vi "Set_Tips_Position_XY.vi"(8 "XYGraph输入":refnum<vi>, 9 "Offset":u8, 10 "Coords":T1, 11 "TipsRef":refnum<vi>) -> ()   [LabVIEW 2015]
uses:
  <vilib>/Utility/miscctls.llb/LVPoint32TypeDef.ctl
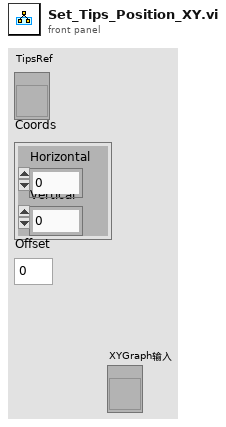
[diagram p1: front panel]
types:
  T1 = typedef "LVPoint32TypeDef.ctl" = cluster{"Horizontal":i32, "Vertical":i32}
  T2 = typedef "LVRectTypeDef.ctl" = cluster{"Left":i16, "Top":i16, "Right":i16, "Bottom":i16}
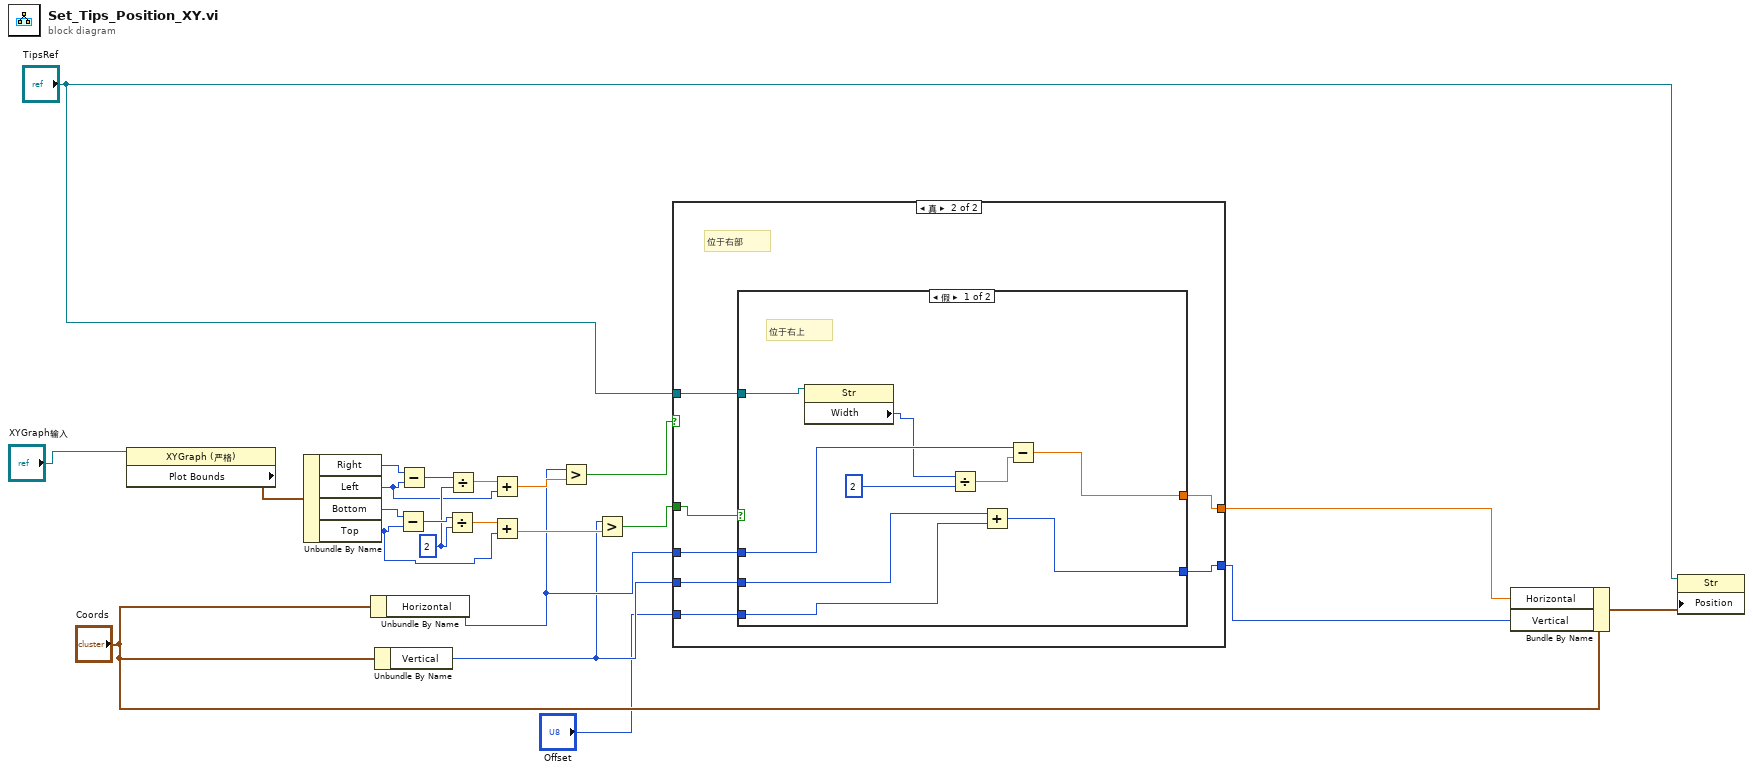
[diagram p0: block diagram]
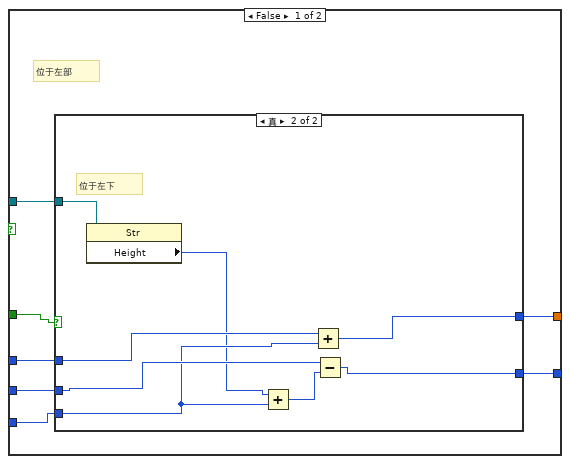
[diagram p2: hidden frame]
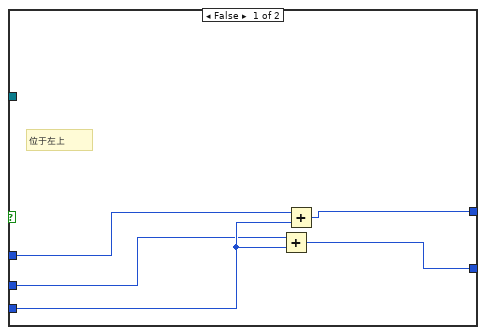
[diagram p3: hidden frame]
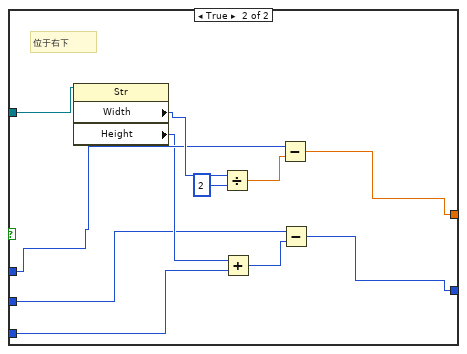
[diagram p4: hidden frame]
diagram:
  w15 = i16 2 ("y")
  n1 = property class="XYGraph (严格)"(reference="XYGraph输入") -> ("Plot Bounds"=w21:T2)  [unwired: 1 in, 2 out]
  n2 = Unbundle By Name(w21) -> ("Right"=w19:i16, "Left"=w13:i16, "Bottom"=w18:i16, "Top"=w11:i16)
  n3 = Unbundle By Name("Coords") -> ("Horizontal"=w6:i32)
  n4 = Unbundle By Name("Coords") -> ("Vertical"=w5:i32)
  n5 = Subtract(x=w18, y=w11) -> (x-y=w17:i16)
  n6 = Subtract(x=w19, y=w13) -> (x-y=w16:i16)
  n7 = Divide(x=w17, y=w15) -> (x/y=w12:dbl)
  n8 = Divide(x=w16, y=w15) -> (x/y=w14:dbl)
  n9 = Add(x=w14, y=w13) -> (x+y=w10:dbl)
  n10 = Add(x=w12, y=w11) -> (x+y=w9:dbl)
  n11 = Greater?(x=w6, y=w10) -> (0:w8:bool)
  n12 = Greater?(x=w5, y=w9) -> (0:w7:bool)
  n13 = case shown="真" w8 {
    tunnel: w7 -> [w30 w50]
    tunnel: w6 -> [w29 w45]
    tunnel: w5 -> [w28 w47]
    tunnel: "Offset" -> [w27 w49]
    tunnel: [w26 w44] -> w3
    tunnel: [w25 w48] -> w2
    tunnel: "TipsRef" -> [w24 w46]
    frame False {
      # "位于左部"
      n14 = case shown="真" w30 {
        tunnel: w29 -> [w35 w43]
        tunnel: w28 -> [w33 w41]
        tunnel: w27 -> [w34 w40]
        tunnel: [w32 w42] -> w26
        tunnel: [w31 w36] -> w25
        tunnel: w24 -> [_ w38]
        frame False {
          # "位于左上"
          n15 = Add(x=w33, y=w34) -> (x+y=w31:i32)
          n16 = Add(x=w35, y=w34) -> (x+y=w32:i32)
        }
        frame True {
          # "位于左下"
          n17 = property class="Str"(reference=w38) -> ("Height"=w37:u32)  [unwired: 1 in, 2 out]
          n18 = Add(x=w37, y=w40) -> (x+y=w39:u32)
          n19 = Add(x=w43, y=w40) -> (x+y=w42:i32)
          n20 = Subtract(x=w41, y=w39) -> (x-y=w36:u32)
        }
      }
    }
    frame True {
      # "位于右部"
      n21 = case shown="假" w50 {
        tunnel: w49 -> [w55 w64]
        tunnel: [w59 w61] -> w48
        tunnel: w47 -> [w58 w62]
        tunnel: w46 -> [w57 w66]
        tunnel: w45 -> [w56 w68]
        tunnel: [w52 w67] -> w44
        frame False {
          # "位于右上"
          n22 = property class="Str"(reference=w57) -> ("Width"=w53:u32)  [unwired: 1 in, 2 out]
          n23 = Divide(x=w53, y=u32 2) -> (x/y=w54:dbl)
          n24 = Add(x=w58, y=w55) -> (x+y=w59:i32)
          n25 = Subtract(x=w56, y=w54) -> (x-y=w52:dbl)
        }
        frame True {
          # "位于右下"
          n26 = property class="Str"(reference=w66) -> ("Width"=w69:u32, "Height"=w63:u32)  [unwired: 1 in, 2 out]
          n27 = Divide(x=w69, y=u32 2) -> (x/y=w70:dbl)
          n28 = Add(x=w63, y=w64) -> (x+y=w65:u32)
          n29 = Subtract(x=w68, y=w70) -> (x-y=w67:dbl)
          n30 = Subtract(x=w62, y=w65) -> (x-y=w61:u32)
        }
      }
    }
  }
  n31 = Bundle By Name(cluster="Coords", "Horizontal"=w3, "Vertical"=w2) -> (w23:T1)
  n32 = property class="Str"(reference="TipsRef", "Position"=w23) -> ()  [unwired: 1 in, 2 out]
